vi "Set Wavelength.vi"(8 "error in (no error)":errorcluster, 10 "wavelength":dbl[unit] min=0.0 max=1.99999e-05 step=1.0000000000000002e-10, 11 "VISA resource name":refnum<visa-resource-name>="COM4") -> (0 "error out":errorcluster, 1 "read buffer":string, 2 "query output":string, 3 "VISA resource name out":refnum<visa-resource-name>)   [LabVIEW 2017]
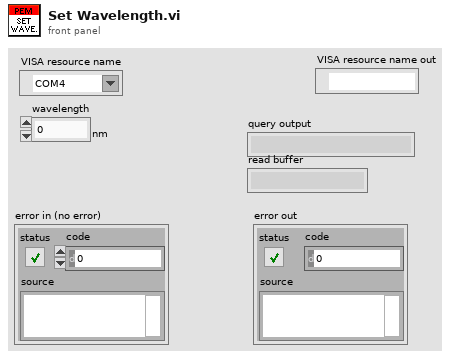
[diagram p1: front panel]
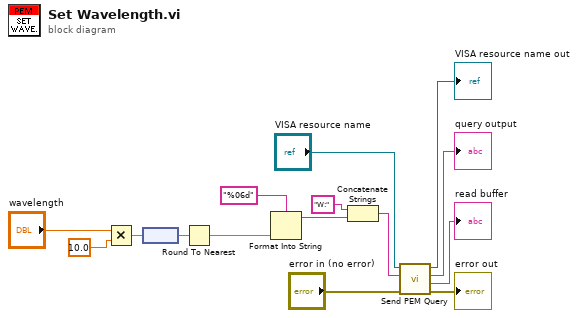
[diagram p0: block diagram]
diagram:
  n1 = Multiply(x="wavelength", y=10.0) -> (x*y=w8:dbl[unit])
  n2 = node(w8) -> (w9:dbl)
  n3 = Round To Nearest(number=w9) -> (nearest integer value=w10:dbl)
  n4 = Format Into String(format string="%06d", w10) -> (resulting string=w13:string)  [unwired: 2 in, 1 out]
  n5 = Concatenate Strings("W:" ("write buffer"), w13) -> (w7:string)
  n6 = call "Send PEM Query.vi"("error in (no error)"="error in (no error)", "query string"=w7, "VISA resource name"="VISA resource name") -> ("error out"=→"error out":errorcluster, "read buffer"=→"read buffer":string, "query output"=→"query output":string, "VISA resource name out"=→"VISA resource name out":refnum<visa-resource-name>)  [unwired: 5 in]
